vi "String History Cacher.vi"(5 "format string":string="%<%H:%M:%S%3u>T", 7 "length":i32=10000, 10 "Include Timestamp(T)":bool=TRUE, 11 "String":string) -> (3 "String Cache":string)   [LabVIEW 2020, in "Communicable State Machine.lvlib"]
doc: "Return the <b>String Cache</b> containing <b>length</b> number of characters, including the new input <b>String</b>.\n\n<b>Inputs:</b>\n - <b>String</b>: History item string\n - <b>length</b>: max history length of cache.\n - <b>Include Timestamp(F)</b>: Include timestamp in the from of every line or not\n\n<b>Outputs:</b>\n - <b>String Cache</b>: The history string"
uses:
  Communicable State Machine.lvlib
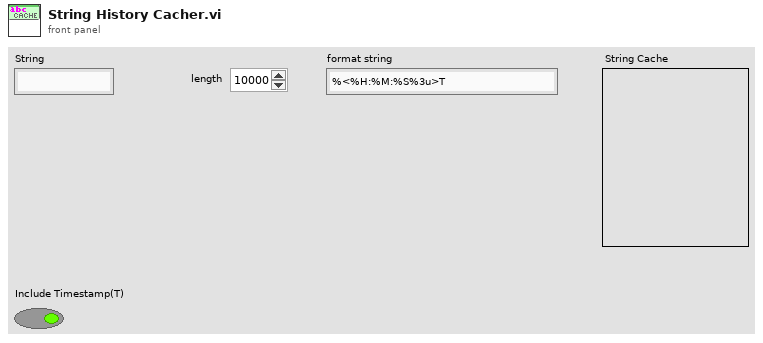
[diagram p1: front panel]
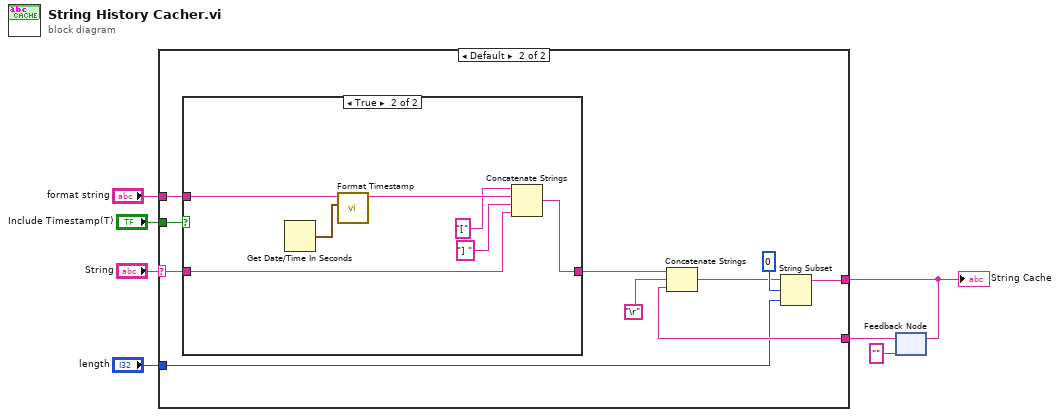
[diagram p0: block diagram]
diagram:
  n1 = feedback #1("") -> (w5:string)
  n2 = case shown="Default" "String" {
    selector: "String" -> [_ w17]
    tunnel: w5 -> [w8 w16]
    tunnel: [w8 w11] -> w3
    tunnel: "Include Timestamp(T)" -> [_ w14]
    tunnel: "length" -> [_ w10]
    tunnel: "format string" -> [_ w9]
    frame "" {
    }
    frame Default {
      n3 = case shown="True" w14 {
        tunnel: w17 -> [w19 w25]
        tunnel: [w19 w24] -> w15
        tunnel: w9 -> [_ w23]
        frame False {
        }
        frame True {
          n4 = Get Date/Time In Seconds() -> (seconds since 1Jan1904=w20:timestamp)
          n5 = call "Format Timestamp.vi"("timestamp"=w20, "format string"=w23) -> ("String"=w22:string)  [unwired: 9 in]
          n6 = Concatenate Strings("[" ("string"), w22, "] " ("string"), w25) -> (w24:string)
        }
      }
      n7 = Concatenate Strings(w15, "\r", w16) -> (w12:string)
      n8 = String Subset(string=w12, offset (0)=0, length (rest)=w10) -> (substring=w11:string)
    }
  }
  "String Cache" <- w3
  n9 = feedback-in #1(w3) -> ()
